vi "Stop Core.vi"(10 "final error code":i32, 11 "Universal Display in":refnum<class "Universal Display.lvclass">) -> (3 "Universal Display out":refnum<class "Universal Display.lvclass">)   [LabVIEW 2013]
doc: "(<B>Filename</B>: Actor Framework.lvlib:Actor.lvclass:Stop Core.vi)\n\nDefines what the actor does before it stops. Use the <B>final error code</B> input to determine whether the actor shut down in response to an error.\n\nBy default, this method does nothing. A descendant class may override it to define behavior, such as shutting down any processes the actor initiated in its override of the Actor Core method."
uses:
  Universal Display.lvclass
panel:
  out "error out":errorcluster
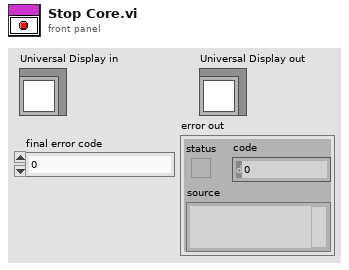
[diagram p1: front panel]
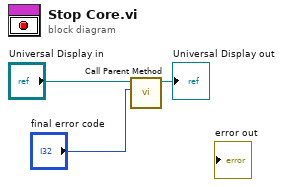
[diagram p0: block diagram]
diagram:
  n1 = call-parent "Call Parent Method"("final error code"="final error code", "Abstract Display in"="Universal Display in") -> ("Abstract Display out"=→"Universal Display out":refnum<class "Universal Display.lvclass">)  [unwired: 9 in]
